vi "Cell Value Constants.vi"() -> (0 "End":T1={"Picture"=3, "Value"=1.0}, 1 "Start":T1={"Picture"=2, "Value"=inf}, 2 "Blocked":T1={"Picture"=1, "Value"=-inf}, 3 "Empty":T1)   [LabVIEW 2019, in "Grassfire Algorithm.lvclass"]
uses:
  Grassfire Algorithm.lvclass
  Solution Grid Cell Private--cluster.ctl
  Solution--picture ring.ctl
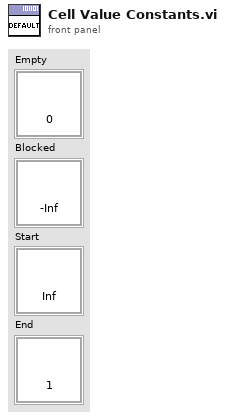
[diagram p1: front panel]
types:
  T1 = typedef "Grassfire Algorithm.lvclass/Solution Grid Cell Private--cluster.ctl" = cluster{"Picture":T2, "Value":dbl}
  T2 = typedef "Grassfire Algorithm.lvclass/Solution--picture ring.ctl" = i64
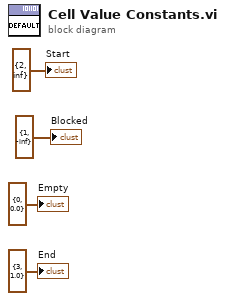
[diagram p0: block diagram]
diagram:
  "Empty" <- T1 {"Picture"=0, "Value"=0.0} ("Empty")
  "Start" <- T1 {"Picture"=2, "Value"=inf} ("Start")
  "Blocked" <- T1 {"Picture"=1, "Value"=-inf} ("Blocked")
  "End" <- T1 {"Picture"=3, "Value"=1.0} ("End")
